vi "Read_Isotope-Table.vi"(8 "error in (no error)":errorcluster, 11 "Standard in":refnum<class "Standard.lvclass">) -> (0 "error out":errorcluster, 2 "Isotope Table":cluster{"isotope":string, "amount cc":dbl}[](array[cluster]), 3 "Standard out":refnum<class "Standard.lvclass">)   [LabVIEW 2018, in "Standard.lvclass"]
uses:
  Standard.lvclass
  Standard.lvclass/Standard.ctl
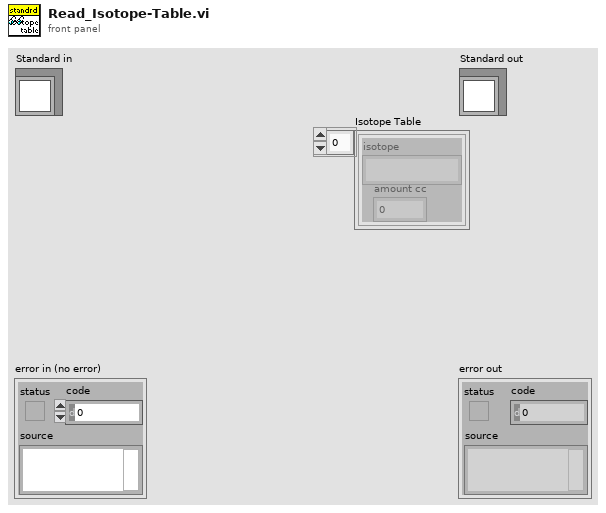
[diagram p1: front panel]
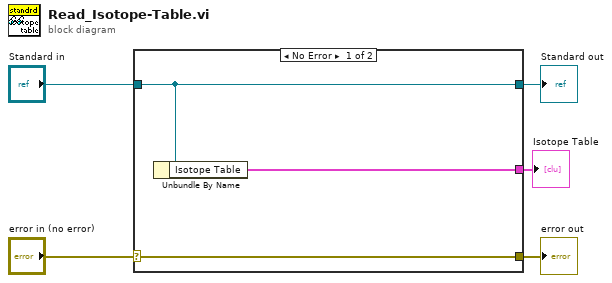
[diagram p0: block diagram]
diagram:
  n1 = case shown="No Error" "error in (no error)" {
    selector: "error in (no error)" -> [w8 w9]
    tunnel: [w8 w9] -> w4
    tunnel: [w7 w10] -> w2
    tunnel: "Standard in" -> [w7 w10]
    tunnel: [w6 _] -> w1
    frame No Error {
      n2 = Unbundle By Name(w7) -> ("Isotope Table"=w6:cluster{"isotope":string, "amount":dbl}[])
    }
    frame Error {
    }
  }
  "error out" <- w4
  "Standard out" <- w2
  "Isotope Table" <- w1
